vi "Toggle Instrument Display.vi"(8 "error in":errorcluster, 9 "Identifier":string, 10 "Panel":i32, 11 "Engine in":refnum<class "Engine.lvclass">) -> (0 "error out":errorcluster, 3 "Engine out":refnum<class "Engine.lvclass">)   [LabVIEW 2023, in "Engine.lvlib" / "Engine.lvclass"]
doc: "<b>override</b> Function to instruct instruments to dock and undock from a user interface panel."
uses:
  Project/Engine.lvclass
  Project/Engine.lvclass/Engine.ctl
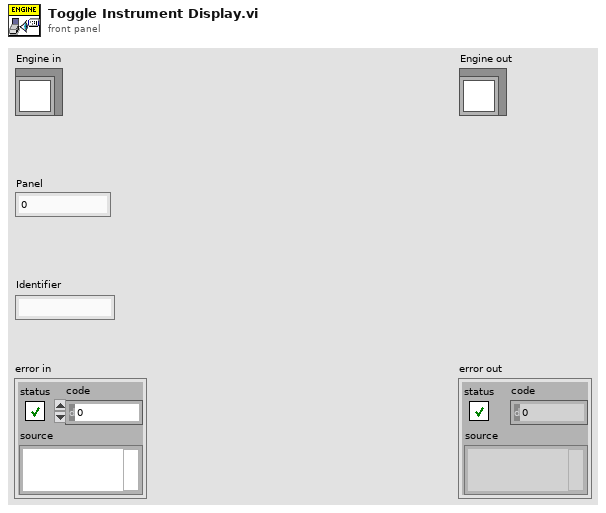
[diagram p1: front panel]
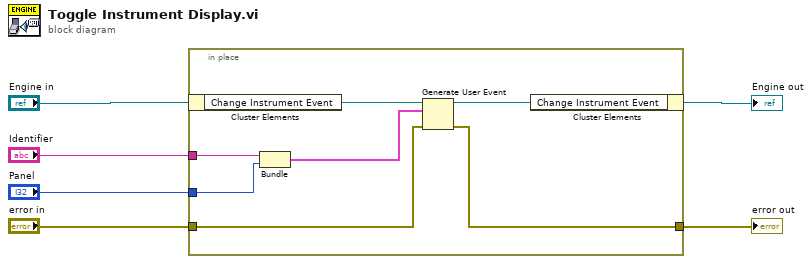
[diagram p0: block diagram]
diagram:
  n1 = in-place {
    in-place-border: "Identifier" -> [w11]
    in-place-border: "Panel" -> [w10]
    in-place-border: "error in" -> [w8]
    in-place-border: [w7] -> w1
    n2 = in-place-cluster #1("Engine in") -> ("Change Instrument Event"=w13:refnum<user-event>)
    n3 = Bundle("Identifier"=w11, "Panel"=w10) -> (w9:cluster{"Identifier":string, "Panel":i32})  [unwired: 1 in]
    n4 = Generate User Event(user event=w13, event data cluster=w9, error in=w8) -> (user event out=w12:refnum<user-event>, error out=w7:errorcluster)  [unwired: 1 in]
    n5 = in-place-cluster #1("Change Instrument Event"=w12) -> (→"Engine out":refnum<class "Engine.lvclass">)
  }
  "error out" <- w1
